vi "Test_WriteUnsignedInteger_ReadCorrectValue.vi"(8 "error in (no error)":errorcluster, 11 "TestCase in":refnum<class "TestMysqlDatabaseConfiguration.lvclass">) -> (0 "error out":errorcluster, 3 "TestCase out":refnum<class "TestMysqlDatabaseConfiguration.lvclass">)   [LabVIEW 2020, in "mysql tests.lvlib" / "TestMysqlDatabaseConfiguration.lvclass"]
uses:
  TestMysqlDatabaseConfiguration.lvclass
  TestMysqlDatabaseConfiguration.lvclass/TestMysqlDatabaseConfiguration.ctl
  <vilib>/gpm_packages/@cs/Configuration/Source/ConfigurationReference/ConfigurationReference.lvclass/ConfigurationReference.ctl
  e002e558-d5e5-459d-ba9e-71d9a5a75879.vi
  1bb3110a-552d-4b56-8dd7-594c2a54aa03.vi
  <vilib>/gpm_packages/@cs/Configuration/Source/ConfigurationReference/Explain DVR Error.vi
  e002e558-d5e5-459d-ba9e-71d9a5a75879.vi/8402ebc0-384b-46ab-989c-700e41096983.vi
  <vilib>/gpm_packages/@cs/Configuration/Source/ConfigurationReference/Read IConfiguration.vi
  <vilib>/gpm_packages/@cs/Configuration/Source/ConfigurationReference/Write IConfiguration.vi
  1bb3110a-552d-4b56-8dd7-594c2a54aa03.vi/7595dcc0-0a31-43e1-86ad-579fe37a7e85.vi
  <vilib>/gpm_packages/@cs/Configuration/Source/IConfiguration/Write U8.vi
  <vilib>/gpm_packages/@cs/Configuration/Source/IConfiguration/Read U8.vi
  <vilib>/gpm_packages/@cs/Configuration/Source/IConfiguration/Read U8.vi/ece91c06-bf80-45f7-8a24-240eaa39dbde.vi
  Source/mysql-queries/mysql-queries.lvclass
  D:/Project/Labview-Projects/database-configuration/Source/IConfigDBQueries/IConfigurationDatabaseQueries.lvclass
  externals/mysql/Source/mysql.net/mysql.lvclass
  D:/Project/Labview-Projects/database-configuration/externals/database-interface/IDatabase/IDatabase/IDatabase.lvclass
  Source/configuration-database.lvclass
  C:/Program Files/National Instruments/LabVIEW 2020/vi.lib/gpm_packages/@cs/Configuration/Source/IConfiguration/IConfiguration.lvclass
  <vilib>/Utility/error.llb/Error Cluster From Error Code.vi
  <vilib>/gpm_packages/@cs/Configuration/Source/IConfiguration/IConfiguration.lvclass
  <vilib>/gpm_packages/@cs/Configuration/Source/ConfigurationReference/ConfigurationReference.lvclass
panel:
  out "Not Found?":bool
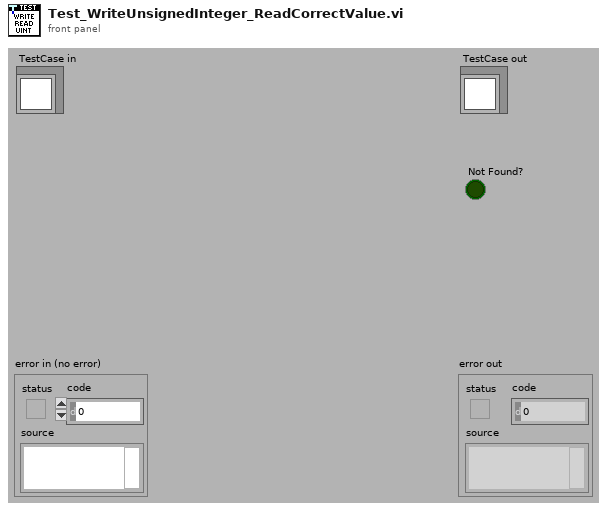
[diagram p1: front panel]
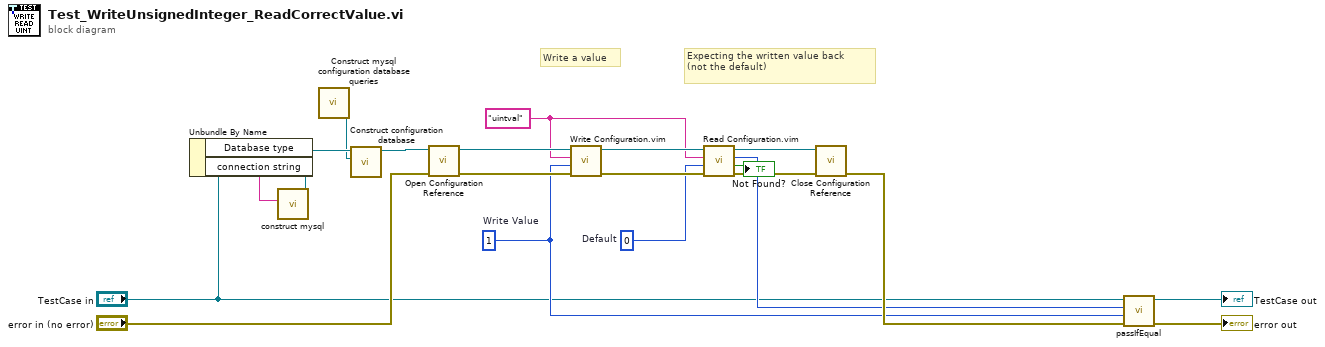
[diagram p0: block diagram]
diagram:
  w12 = u8 0  # Default
  w7 = u8 1  # Write Value
  w13 = "uintval" ("Name")
  # "Write a value"
  # "Expecting the written value back\n(not the default)"
  n1 = Unbundle By Name("TestCase in") -> ("connection string"=w4:string)  [unwired: 1 out]
  n2 = call "construct mysql.vi"("Connection string"=w4) -> ("mysql out"=w3:refnum<class "mysql.lvclass">)  [unwired: 9 in, 1 out]
  n3 = call "Construct mysql configuration database queries.vi"() -> ("mysql-configdb-queries out"=w2:refnum<class "mysql-queries.lvclass">)  [unwired: 10 in, 1 out]
  n4 = call "Construct configuration database.vi"("SQL logic type"=w2, "Database type in"=w3) -> ("database-configuration out"=w6:refnum<class "configuration-database.lvclass">)  [unwired: 8 in, 1 out]
  n5 = call <vilib>:"Open Configuration Reference.vi"("error in (no error)"="error in (no error)", "Configuration Type"=w6) -> ("error out"=w14:errorcluster, "Configuration Reference"=w15:refnum<data-value>)  [unwired: 8 in]
  n6 = call "Write Configuration.vim"("error in (no error)"=w14, "Value"=w7, "Name"=w13, "Configuration Reference in"=w15) -> ("error out"=w16:errorcluster, "Configuration Reference out"=w17:refnum<data-value>)  [unwired: 6 in]
  n7 = call "Read Configuration.vim"("error in (no error)"=w16, "Type (Default Value If Not Found)"=w12, "Name"=w13, "Configuration Reference in"=w17) -> ("error out"=w10:errorcluster, "Not Found?"=→"Not Found?":bool, "Value"=w8:u8, "Configuration Reference out"=w11:refnum<data-value>)  [unwired: 4 in]
  n8 = call <vilib>:"Close Configuration Reference.vi"("error in (no error)"=w10, "Configuration Reference"=w11) -> ("error out"=w9:errorcluster)  [unwired: 9 in]
  n9 = call-dynamic "passIfEqual.vi"("error in (no error)"=w9, "y"=w7, "x"=w8, "TestCase in"="TestCase in") -> ("error out"=→"error out":errorcluster, "TestCase out"=→"TestCase out":refnum<class "TestMysqlDatabaseConfiguration.lvclass">)  [unwired: 6 in]
